vi "Taller 1 punto 5.vi"() -> ()   [LabVIEW 2017]
panel:
  in  "Dirección":bool
  out "Tope Derecho":bool
  out "Tope Izquierdo":bool
  out "Banda":dbl(slide) scale=0.0..1200.0
  in  "stop":bool
  in  "Velocidad (m/300ms)":dbl(knob) scale=0.0..10.0
  in  "Acción":bool
  # "TALLER 1, PUNTO 5\nLUZ ANDREA JARAMILLO CASTILLO"
  # "Continuar"
  # "Derecha"
  # "Izquierda"
  # "Detener"
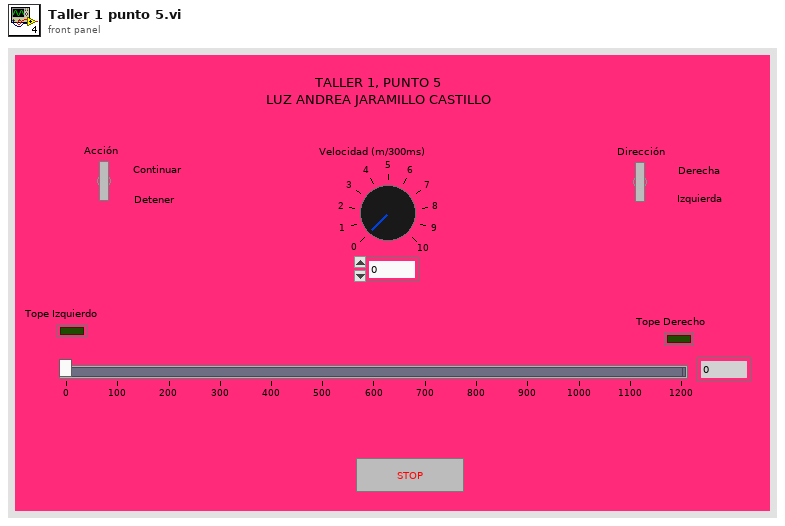
[diagram p1: front panel]
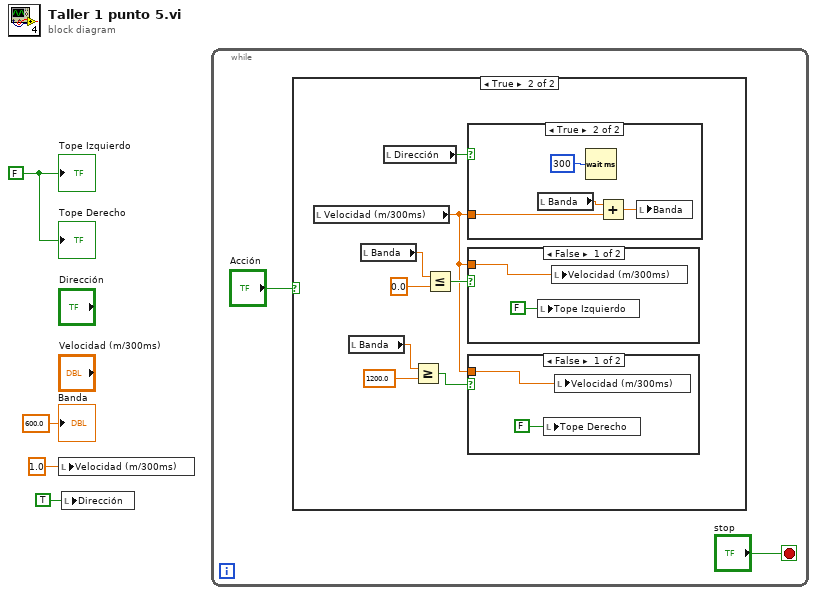
[diagram p0: block diagram]
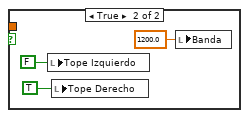
[diagram p3: hidden frame]
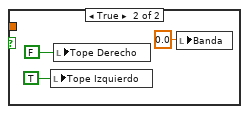
[diagram p4: hidden frame]
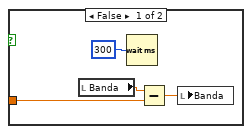
[diagram p5: hidden frame]
diagram:
  w1 = FALSE ("Tope Izquierdo")
  n1 = local write "Velocidad (m/300ms)"(1.0 ("Velocidad (m/300ms)")) -> ()
  n2 = local write "Dirección"(TRUE ("Dirección")) -> ()
  n3 = while {
    stop <- "stop" stop-if-true
    n4 = case shown="True" "Acción" {
      frame False {
      }
      frame True {
        n5 = local read "Velocidad (m/300ms)"() -> (w8:dbl)
        n6 = local read "Banda"() -> (w12:dbl)
        n7 = local read "Banda"() -> (w7:dbl)
        n8 = local read "Dirección"() -> (w14:bool)
        n9 = Greater Or Equal?(x=w12, y=1200.0) -> (x >= y?=w9:bool)
        n10 = Less Or Equal?(x=w7, y=0.0) -> (x <= y?=w10:bool)
        n11 = case shown="True" w14 {
          tunnel: w8 -> [w26 w29]
          frame False {
            n12 = local read "Banda"() -> (w25:dbl)
            n13 = Wait (ms)(milliseconds to wait=u32 300) -> ()  [unwired: 1 out]
            n14 = Subtract(x=w25, y=w26) -> (x-y=w28:dbl)
            n15 = local write "Banda"(w28) -> ()
          }
          frame True {
            n16 = local read "Banda"() -> (w32:dbl)
            n17 = Wait (ms)(milliseconds to wait=u32 300) -> ()  [unwired: 1 out]
            n18 = Add(x=w32, y=w29) -> (x+y=w31:dbl)
            n19 = local write "Banda"(w31) -> ()
          }
        }
        n20 = case shown="False" w10 {
          tunnel: w8 -> [w21 _]
          frame False {
            n21 = local write "Tope Izquierdo"(FALSE ("Dirección")) -> ()
            n22 = local write "Velocidad (m/300ms)"(w21) -> ()
          }
          frame True {
            n23 = local write "Tope Izquierdo"(TRUE ("Dirección")) -> ()
            n24 = local write "Tope Derecho"(FALSE ("Dirección")) -> ()
            n25 = local write "Banda"(0.0 ("Banda")) -> ()
          }
        }
        n26 = case shown="False" w9 {
          tunnel: w8 -> [w16 _]
          frame False {
            n27 = local write "Tope Derecho"(FALSE ("Dirección")) -> ()
            n28 = local write "Velocidad (m/300ms)"(w16) -> ()
          }
          frame True {
            n29 = local write "Tope Izquierdo"(FALSE ("Dirección")) -> ()
            n30 = local write "Tope Derecho"(TRUE ("Dirección")) -> ()
            n31 = local write "Banda"(1200.0 ("Banda")) -> ()
          }
        }
      }
    }
  }
  "Banda" <- 600.0 ("Banda")
  "Tope Izquierdo" <- w1
  "Tope Derecho" <- w1
